vi "Trim Null Array.vi"(11 "String":string="<!DOCTYPE HTML PUBLIC \"-//W3C//DTD HTML 4.01//EN\" \"http://www.w3.org/TR/html4/strict.dtd\"><html><head><link rel=\"shortcut icon\" href=\"//ssl.gstatic.com/docs/spreadsheets/forms/favicon_jfk.png\" type=\"image/x-icon\">\n<meta http-equiv=\"Content-type\" content=\"text/html; charset=utf-8\">\n<title>demo1</title>\n\n<link href='/static/spreadsheets/client/css/779923916-published_form_compiled.css' type='text/css' rel='stylesheet'>\n</head>\n<body class=\"ss-base-body\" dir=\"ltr\" itemscope itemtype=\"http://schema.org/CreativeWork/FormObject\">\n\n<div class=\"ss-form-container\">\n<div class=\"ss-form-heading\"><h1 class=\"ss-form-title\">demo1</h1>\n<p></p>\n\n\n<hr class=\"ss-email-break\" style=\"display:none;\">\n</div>\n<div class=\"ss-form\"><form action=\"https://docs.google.com/spreadsheet/formResponse?formkey=dFNhUnAta3JpbUNkdlNvUmFVeTFBdVE6MQ&amp;ifq\" method=\"POST\" id=\"ss-form\">\n\n<br>\n<div class=\"errorbox-good\">\n<div class=\"ss-item  ss-text\"><div class=\"ss-form-entry\"><label class=\"ss-q-title\" for=\"entry_0\">x\n</label>\n<label class=\"ss-q-help\" for=\"entry_0\"></label>\n<input type=\"text\" name=\"entry.0.single\" value=\"\" class=\"ss-q-short\" id=\"entry_0\"></div></div></div>\n<br> <div class=\"errorbox-good\">\n<div class=\"ss-item  ss-text\"><div class=\"ss-form-entry\"><label class=\"ss-q-title\" for=\"entry_1\">y\n</label>\n<label class=\"ss-q-help\" for=\"entry_1\"></label>\n<input type=\"text\" name=\"entry.1.single\" value=\"\" class=\"ss-q-short\" id=\"entry_1\"></div></div></div>\n<br> <div class=\"errorbox-good\">\n<div class=\"ss-item  ss-text\"><div class=\"ss-form-entry\"><label class=\"ss-q-title\" for=\"entry_2\">z\n</label>\n<label class=\"ss-q-help\" for=\"entry_2\"></label>\n<input type=\"text\" name=\"entry.2.single\" value=\"\" class=\"ss-q-short\" id=\"entry_2\"></div></div></div>\n<br> <div class=\"errorbox-good\">\n<div class=\"ss-item  ss-text\"><div class=\"ss-form-entry\"><label class=\"ss-q-title\" for=\"entry_4\">1\n</label>\n<label class=\"ss-q-help\" for=\"entry_4\"></label>\n<input type=\"text\" name=\"entry.4.single\" value=\"\" class=\"ss-q-short\" id=\"entry_4\"></div></div></div>\n<br> <div class=\"errorbox-good\">\n<div class=\"ss-item  ss-text\"><div class=\"ss-form-entry\"><label class=\"ss-q-title\" for=\"entry_6\">2\n</label>\n<label class=\"ss-q-help\" for=\"entry_6\"></label>\n<input type=\"text\" name=\"entry.6.single\" value=\"\" class=\"ss-q-short\" id=\"entry_6\"></div></div></div>\n<br> <div class=\"errorbox-good\">\n<div class=\"ss-item  ss-text\"><div class=\"ss-form-entry\"><label class=\"ss-q-title\" for=\"entry_8\">3\n</label>\n<label class=\"ss-q-help\" for=\"entry_8\"></label>\n<input type=\"text\" name=\"entry.8.single\" value=\"\" class=\"ss-q-short\" id=\"entry_8\"></div></div></div>\n<br>\n<input type=\"hidden\" name=\"pageNumber\" value=\"0\">\n<input type=\"hidden\" name=\"backupCache\" value=\"\">\n\n\n<div class=\"ss-item ss-navigate\"><div class=\"ss-form-entry\">\n<input type=\"submit\" name=\"submit\" value=\"Submit\"></div></div></form>\n<script type=\"text/javascript\">\n      \n      (function() {\nvar divs = document.getElementById('ss-form').\ngetElementsByTagName('div');\nvar numDivs = divs.length;\nfor (var j = 0; j < numDivs; j++) {\nif (divs[j].className == 'errorbox-bad') {\ndivs[j].lastChild.firstChild.lastChild.focus();\nreturn;\n}\n}\nfor (var i = 0; i < numDivs; i++) {\nvar div = divs[i];\nif (div.className == 'ss-form-entry' &&\ndiv.firstChild &&\ndiv.firstChild.className == 'ss-q-title') {\ndiv.lastChild.focus();\nreturn;\n}\n}\n})();\n      </script></div>\n<div class=\"ss-footer\"><div class=\"ss-attribution\"></div>\n<div class=\"ss-legal\"><span class=\"ss-powered-by\">Powered by <a href=\"http://docs.google.com\">Google Docs</a></span>\n<span class=\"ss-terms\"><small><a href=\"https://docs.google.com/spreadsheet/reportabuse?formkey=dFNhUnAta3JpbUNkdlNvUmFVeTFBdVE6MQ&amp;source=https%253A%252F%252Fdocs.google.com%252Fspreadsheet%252Fviewform%253Fformkey%253DdFNhUnAta3JpbUNkdlNvUmFVeTFBdVE6MQ\">Report Abuse</a>\n-\n<a href=\"http://www.google.com/accounts/TOS\">Terms of Service</a>\n-\n<a href=\"http://www.google.com/google-d-s/terms.html\">Additional Terms</a></small></span></div></div></div></body></html>") -> (3 "output array":string[](array[string]))   [LabVIEW 2011]
panel:
  out "Array":string[](array[string])
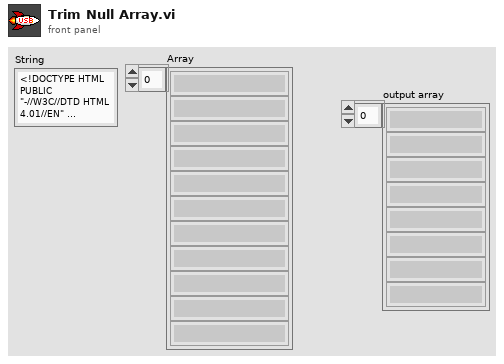
[diagram p1: front panel]
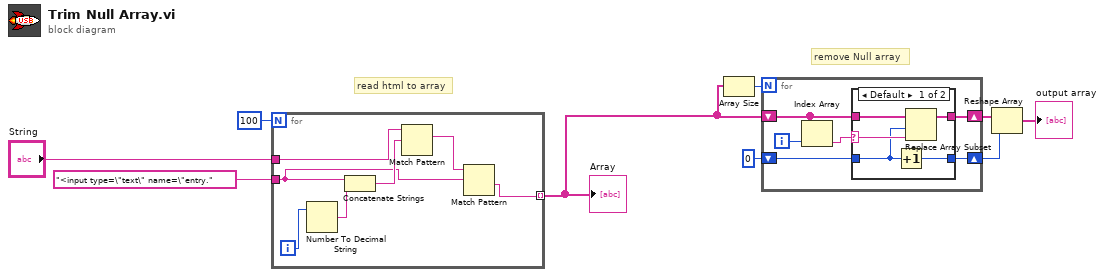
[diagram p0: block diagram]
diagram:
  # "read html to array"
  # "remove Null array"
  n1 = for {
    N: 100 -> [_]
    tunnel: "String" -> [w15]
    tunnel: "<input type=\"text\" name=\"entry." -> [w12]
    tunnel: [w10] -> w2 mode=indexing
    i -> [w11]
    n2 = Number To Decimal String(number=w11) -> (decimal integer string=w16:string)  [unwired: 1 in]
    n3 = Concatenate Strings(w12, w16) -> (w14:string)
    n4 = Match Pattern(string=w15, regular expression=w14) -> (match substring=w13:string)  [unwired: 1 in, 3 out]
    n5 = Match Pattern(string=w13, regular expression=w12) -> (after substring=w10:string)  [unwired: 1 in, 3 out]
  }
  "Array" <- w2
  n6 = Array Size(array=w2) -> (size(s)=w6:i32)
  n7 = for {
    N: w6 -> [_]
    shift-right: [w22] -> w5
    shift-left: w2 -> [w21]
    shift-right: [w18] -> w3
    shift-left: 0 -> [w17]
    i -> [w19]
    n8 = Index Array(array=w21, index=w19) -> (element=w20:string)
    n9 = case shown="Default" w20 {
      selector: w20 -> [w25 _]
      tunnel: w21 -> [w27 w28]
      tunnel: [w26 w28] -> w22
      tunnel: [w23 w29] -> w18
      tunnel: w17 -> [w24 w29]
      frame Default {
        n10 = Increment(x=w24) -> (x+1=w23:i32)
        n11 = Replace Array Subset(array=w27, new element=w25, index=w24) -> (w26:string[])
      }
      frame "" {
      }
    }
  }
  n12 = Reshape Array(w5, w3) -> (→"output array":string[])
